vi "GEOM_template2keys.vi"(8 "error in (no error)":errorcluster, 11 "file":path) -> (0 "error out":errorcluster, 1 "header template":path, 2 "number of keywords found":i32, 3 "HeaderModules":T1[](array[typedef]))   [LabVIEW 2016]
doc: "This VI reads the configuration file searching for the \"infofile\" keyword. Then, it goes and reads the specified file, which should be a template for the TCS info format"
uses:
  GEOM_HeaderModule.ctl
  <vilib>/Utility/config.llb/Read Key (String).vi
  <vilib>/Utility/config.llb/NI_LVConfig.lvlib
panel:
  in  "default hdr file":path=path "/home/arcconfig/GEOM_INFO.tpl"
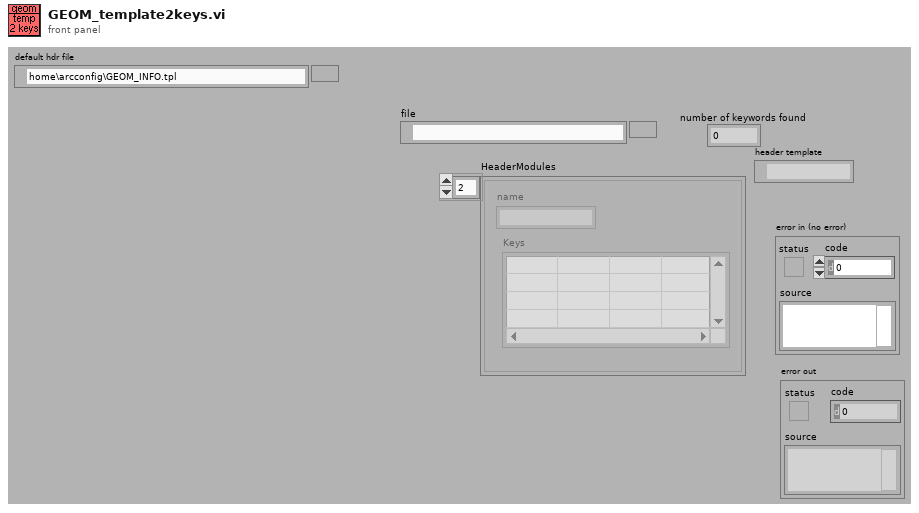
[diagram p1: front panel]
types:
  T1 = typedef "GEOM_HeaderModule.ctl" = cluster{"name":string, "Keys":string[][]}
  T2 = typedef "NI_LVConfig.lvlib/Config Data RefNum.ctl" = refnum<k1>
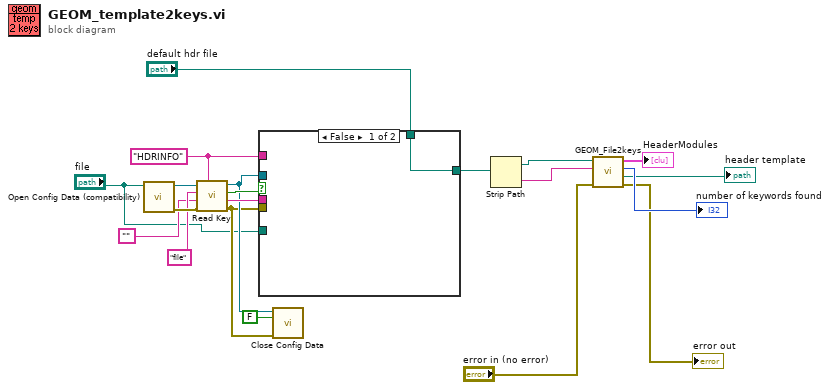
[diagram p0: block diagram]
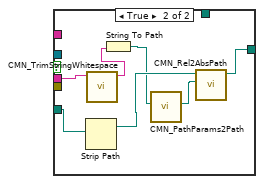
[diagram p2: hidden frame]
diagram:
  w14 = "HDRINFO" ("section")
  n1 = call <vilib>:"Open Config Data (compatibility).vi"("configuration file path"="file") -> ("error out"=w19:errorcluster, "refnum"=w20:T2)  [unwired: 8 in, 1 out]
  n2 = call-poly <vilib>:"Read Key.vi"("section"=w14, "error in (no error)"=w19, "default value"="", "key"="file", "refnum"=w20) -> ("error out"=w11:errorcluster, "value"=w15:string, "found?"=w16:bool, "refnum out"=w12:T2)  [unwired: 1 in, 2 out]
  n3 = case shown="False" w16 {
    tunnel: w15 -> [_ w28]
    tunnel: [w21 w26] -> w3
    tunnel: w12 -> [_ _]
    tunnel: w11 -> [_ _]
    tunnel: w14 -> [_ _]
    tunnel: "default hdr file" -> [w21 _]
    tunnel: "file" -> [_ w24]
    frame False {
    }
    frame True {
      n4 = Strip Path(path=w24) -> (stripped path=w25:path)  [unwired: 1 out]
      n5 = call "CMN_TrimStringWhitespace.vi"("string"=w28) -> ("trimmed string"=w27:string)  [unwired: 1 in, 8 out]
      n6 = String To Path(string=w27) -> (path=w23:path)
      n7 = call "CMN_PathParams2Path.vi"("Path In"=w23) -> ("Path out"=w22:path)  [unwired: 2 in, 8 out]
      n8 = call "CMN_Rel2AbsPath.vi"("test path"=w22, "absolute path"=w25) -> ("output path"=w26:path)  [unwired: 1 in, 8 out]
    }
  }
  n9 = call <vilib>:"Close Config Data.vi"("error in (no error)"=w11, "write file if changed (T)"=FALSE ("write configuration file? (T)"), "refnum"=w12) -> ()  [unwired: 9 out]
  n10 = Strip Path(path=w3) -> (stripped path=w2:path, name=w1:string)
  n11 = call "GEOM_File2keys.vi"("error in (no error)"="error in (no error)", "template in"=w1, "ref dir"=w2) -> ("error out"=→"error out":errorcluster, "header template"=→"header template":path, "number of keywords found"=→"number of keywords found":i32, "HeaderModules"=→"HeaderModules":T1[])  [unwired: 5 out]
